vi "Kaelus PIM Measure Samples.vi"(8 "error in (no error)":errorcluster) -> (0 "error out":errorcluster, 3 "Measurement Results":T1 {"IMPower_dBc(s)" format="%.2f"; "TxFreqs" format="%.2f"; "IMFreq(s)" format="%.2f"; "IMPower(s)" format="%.2f"; "TxPower" format="%.2f"})   [LabVIEW 2011]
uses:
  PIM Results.ctl
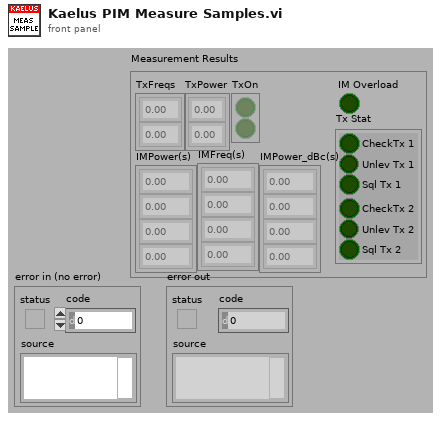
[diagram p1: front panel]
types:
  T1 = typedef "PIM Results.ctl" = cluster{"TxFreqs":dbl[], "TxPower":dbl[], "TxOn":bool[], "IMPower(s)":dbl[], "IMFreq(s)":dbl[], "Tx Stat":cluster{"CheckTx 1":bool, "Unlev Tx 1":bool, "Sql Tx 1":bool, "CheckTx 2":bool, "Unlev Tx 2":bool, "Sql Tx 2":bool}, "IM Overload":bool, "IMPower_dBc(s)":dbl[]}
  T2 = typedef "PIM.API.Command.Unique.ctl" = cluster{"#attributes":cluster{"Action":string}, "Double":dbl[], "Integer":i32[], "Boolean":bool[], "String":string[]}
  T3 = typedef "PIM.API.Response.Unique.ctl" = cluster{"#attributes":cluster{"Action":string, "Units":string}, "Double":dbl[], "Integer":i32[], "Boolean":bool[], "String":string[], "Sample":T4[], "Status":cluster{"#attributes":cluster{"Error":bool, "Code":i32}, "Message":string}[]}
  T4 = typedef "PIM.API.Response.Samples.ctl" = cluster{"TX1":cluster{"#attributes":cluster{"Frequency":dbl, "Power_dBm":dbl, "Power_Watts":dbl, "CheckTx":bool, "Unleveled":bool, "Squelched":bool, "Temperature":dbl, "ToneOn":bool}}, "TX2":cluster{"#attributes":cluster{"Frequency":dbl, "Power_dBm":dbl, "Power_Watts":dbl, "CheckTx":bool, "Unleveled":bool, "Squelched":bool, "Temperature":dbl, "ToneOn":bool}}, "IM":cluster{"#attributes":cluster{"Frequency":dbl, "Power_dBm":dbl, "PeakPower_dBm":dbl, "Power_dBc":dbl, "PeakPower_dBc":dbl, "IM_Order":u8, "IM Overload":bool}}[], "#attributes":cluster{"Count":u32, "Total":u32, "Finished?":bool, "Sweep Leg":T5, "F1":dbl, "F2":dbl, "FStep":dbl}}
  T5 = typedef "iQA Sweep Behavior.ctl" = enum16{"F2Down", "F1Up", "RxMultiIM"}
  T6 = cluster{"#attributes":cluster{"Frequency":dbl, "Power_dBm":dbl, "PeakPower_dBm":dbl, "Power_dBc":dbl, "PeakPower_dBc":dbl, "IM_Order":u8, "IM Overload":bool}}[]
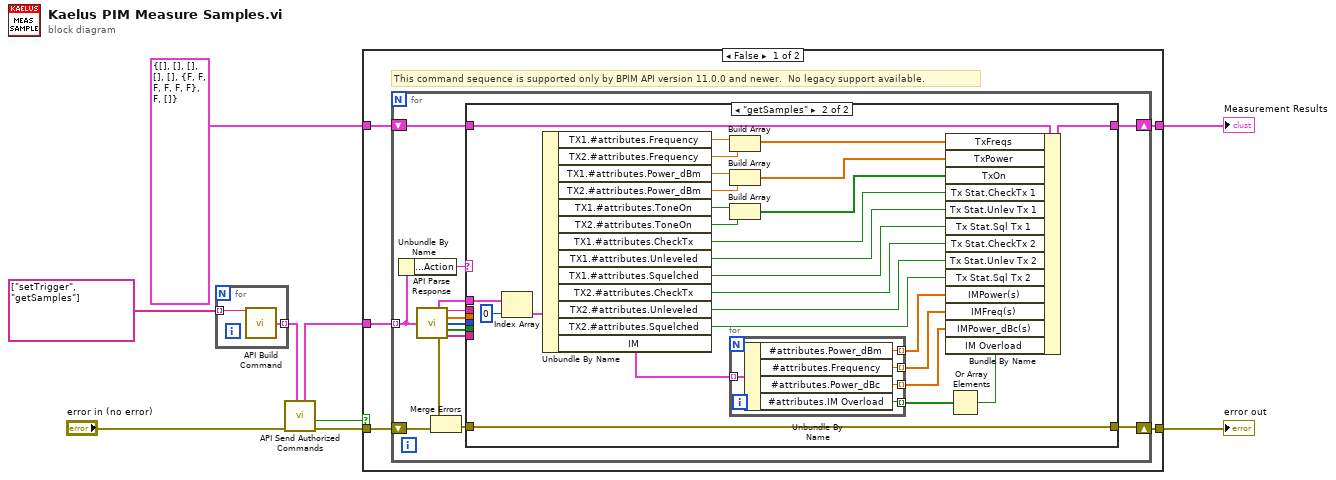
[diagram p0: block diagram]
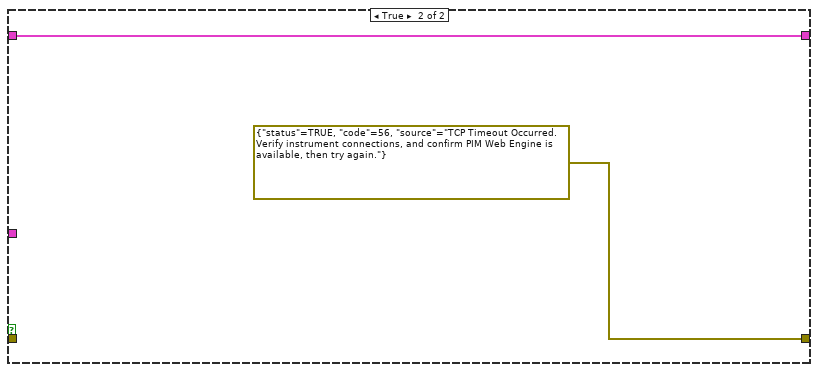
[diagram p3: hidden frame]
diagram:
  n1 = for {
    tunnel: string[] ["setTrigger", "getSamples"] -> [w11] mode=indexing
    tunnel: [w10] -> w4 mode=indexing
    n2 = call "API Build Command.vi"("Action"=w11) -> ("PIM.API.Command.Unique"=w10:T2)  [unwired: 14 in]
  }
  n3 = call "API Send Authorized Commands.vi"("Commands"=w4, "error in (no error)"="error in (no error)") -> ("error out"=w3:errorcluster, "Timed Out?"=w1:bool, "Responses"=w2:T3[])  [unwired: 7 in]
  n4 = case shown="False" w1 {
    tunnel: T1 {"TxFreqs"=[], "TxPower"=[], "TxOn"=[], "IMPower(s)"=[], "IMFreq(s)"=[], "Tx Stat"={"CheckTx 1"=FALSE, "Unlev Tx 1"=FALSE, "Sql Tx 1"=FALSE, "CheckTx 2"=FALSE, "Unlev Tx 2"=FALSE, "Sql Tx 2"=FALSE}, "IM Overload"=FALSE, "IMPower_dBc(s)"=[]} ("Measurement Results") -> [w16 w65]
    tunnel: [w15 w65] -> w7
    tunnel: [w14 errorcluster {"status"=TRUE, "code"=56, "source"="TCP Timeout Occurred.  Verify instrument connections, and confirm PIM Web Engine is available, then try again."} ("error out")] -> w5
    tunnel: w3 -> [w13 _]
    tunnel: w2 -> [w12 _]
    frame False {
      # "This command sequence is supported only by BPIM API version 11.0.0 and newer.  No legacy support available."
      n5 = for {
        shift-right: [w22] -> w14
        shift-left: w13 -> [w20]
        tunnel: w12 -> [w28] mode=indexing
        shift-right: [w18] -> w15
        shift-left: w16 -> [w29]
        n6 = Unbundle By Name(w28) -> ("#attributes.Action"=w30:string)
        n7 = call "API Parse Response.vi"("PIM.API.Response.Unique"=w28) -> ("Sample"=w17:T4[], "Action"=w27:string, "Double"=w26:dbl[], "Integer"=w25:i32[], "Boolean"=w24:bool[], "error out"=w21:errorcluster, "String"=w23:string[])  [unwired: 8 in]
        n8 = Merge Errors(w21, w20) -> (w19:errorcluster)
        n9 = case shown="\"getSamples\"" w30 {
          tunnel: w29 -> [w32 w59]
          tunnel: [w32 w58] -> w18
          tunnel: [w31 w57] -> w22
          tunnel: w27 -> [_ _]
          tunnel: w26 -> [_ _]
          tunnel: w25 -> [_ _]
          tunnel: w24 -> [_ _]
          tunnel: w23 -> [_ _]
          tunnel: w19 -> [w31 w57]
          tunnel: w17 -> [_ w56]
          frame "SetTrigger", Default {
            # "No Data to be set here"
          }
          frame "getSamples" {
            n10 = Index Array(array=w56, index=0) -> (element=w54:T4)
            n11 = Unbundle By Name(w54) -> ("TX1.#attributes.Frequency"=w53:dbl, "TX2.#attributes.Frequency"=w48:dbl, "TX1.#attributes.Power_dBm"=w52:dbl, "TX2.#attributes.Power_dBm"=w51:dbl, "TX1.#attributes.ToneOn"=w50:bool, "TX2.#attributes.ToneOn"=w49:bool, "TX1.#attributes.CheckTx"=w39:bool, "TX1.#attributes.Unleveled"=w40:bool, "TX1.#attributes.Squelched"=w41:bool, "TX2.#attributes.CheckTx"=w42:bool, "TX2.#attributes.Unleveled"=w43:bool, "TX2.#attributes.Squelched"=w44:bool, "IM"=w38:T6)
            n12 = Build Array(w53, w48) -> (w47:dbl[])
            n13 = Build Array(w52, w51) -> (w46:dbl[])
            n14 = Build Array(w50, w49) -> (w45:bool[])
            n15 = for {
              tunnel: [w64] -> w35 mode=indexing
              tunnel: [w63] -> w36 mode=indexing
              tunnel: [w62] -> w37 mode=indexing
              tunnel: w38 -> [w61] mode=indexing
              tunnel: [w60] -> w34 mode=indexing
              n16 = Unbundle By Name(w61) -> ("#attributes.Power_dBm"=w62:dbl, "#attributes.Frequency"=w63:dbl, "#attributes.Power_dBc"=w64:dbl, "#attributes.IM Overload"=w60:bool)
            }
            n17 = Or Array Elements(Boolean array=w34) -> (logical OR=w33:bool)
            n18 = Bundle By Name(cluster=w59, "TxFreqs"=w47, "TxPower"=w46, "TxOn"=w45, "Tx Stat.CheckTx 1"=w39, "Tx Stat.Unlev Tx 1"=w40, "Tx Stat.Sql Tx 1"=w41, "Tx Stat.CheckTx 2"=w42, "Tx Stat.Unlev Tx 2"=w43, "Tx Stat.Sql Tx 2"=w44, "IMPower(s)"=w37, "IMFreq(s)"=w36, "IMPower_dBc(s)"=w35, "IM Overload"=w33) -> (w58:T1)
          }
        }
      }
    }
    frame True {
    }
  }
  "Measurement Results" <- w7
  "error out" <- w5
